vi "DT_Get_All_DependencyFileList.vi"(7 "Framwork Type":T1) -> (1 "rel. Filepaths .js":path[](array[path]), 2 "rel. Filepaths .css":path[](array[path]))   [LabVIEW 2014]
uses:
  controls/StylingFrameworks_Enum.ctl
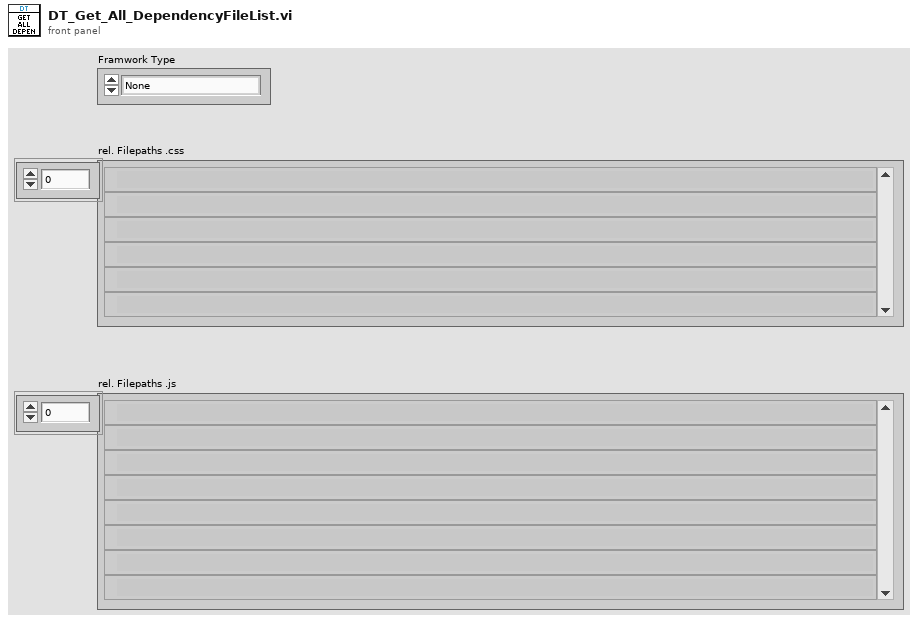
[diagram p1: front panel]
types:
  T1 = typedef "StylingFrameworks_Enum.ctl" = enum16{"None", "Bootstrap4", "Semantic-UI", "Custom"}
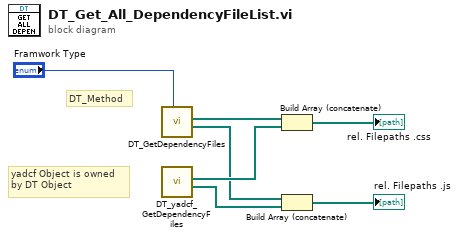
[diagram p0: block diagram]
diagram:
  # "yadcf Object is owned\nby DT Object"
  # "DT_Method"
  n1 = call "DT_GetDependencyFiles.vi"("Framwork Type"="Framwork Type") -> ("rel. Filepaths .js"=w2:path[], "rel. Filepaths .css"=w6:path[])  [unwired: 9 in]
  n2 = call "DT_yadcf_GetDependencyFiles.vi"() -> ("rel. Filepaths .js"=w1:path[], "rel. Filepaths .css"=w3:path[])  [unwired: 10 in]
  n3 = Build Array (concatenate)(w6, w3) -> (→"rel. Filepaths .css":path[])
  n4 = Build Array (concatenate)(w2, w1) -> (→"rel. Filepaths .js":path[])
